vi "Configure Setpoint 1.vi"(5 "Retry Attempts (0)":i32 min=0, 7 "Unit Address (-1)":i32=-1, 8 "error in (no error)":errorcluster, 10 "Setpoint value":dbl format="%#_13g", 11 "VISA resource name (in)":refnum<visa-resource-name>) -> (0 "error out":errorcluster, 2 "Response Cluster":T1 {"Command ID" format="%x"}, 3 "VISA resource name (out)":refnum<visa-resource-name>)   [LabVIEW 2020, in "Omega Platinum Series.lvlib"]
doc: "Configures setpoint 1."
uses:
  <instrlib>/RxnRover/OmegaPlatinumSeriesDriver/Omega Platinum Series.lvlib
  <instrlib>/RxnRover/OmegaPlatinumSeriesDriver/Public/Type Defs/Response.ctl
panel:
  out "Command":string
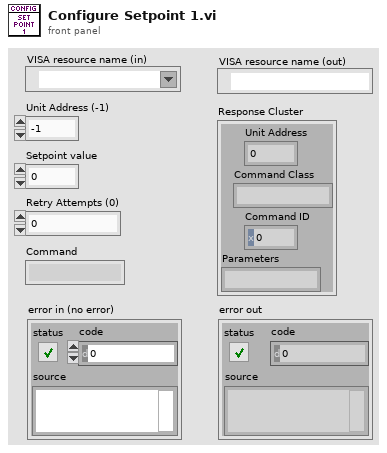
[diagram p1: front panel]
types:
  T1 = typedef "Omega Platinum Series.lvlib/Response.ctl" = cluster{"Unit Address":i32, "Command Class":string, "Command ID":u32, "Parameters":string}
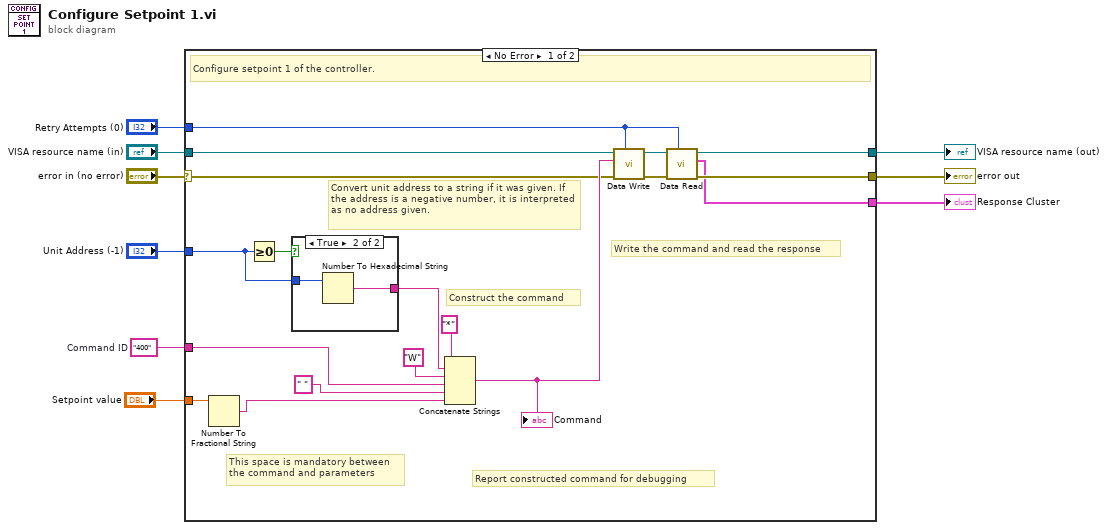
[diagram p0: block diagram]
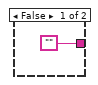
[diagram p2: hidden frame]
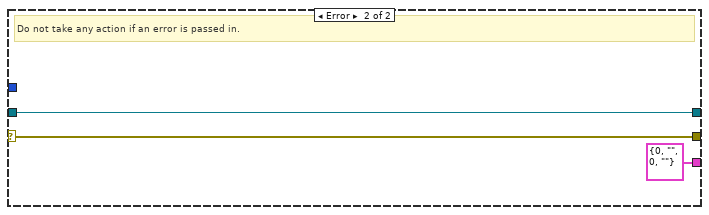
[diagram p3: hidden frame]
diagram:
  w9 = "400"  # Command ID
  n1 = case shown="No Error" "error in (no error)" {
    selector: "error in (no error)" -> [w21 w33]
    tunnel: w9 -> [w14 _]
    tunnel: "Unit Address (-1)" -> [w25 _]
    tunnel: [w17 w33] -> w6
    tunnel: "VISA resource name (in)" -> [w23 w32]
    tunnel: [w18 w32] -> w4
    tunnel: [w16 T1 {"Unit Address"=0, "Command Class"="", "Command ID"=0, "Parameters"=""} ("Response Cluster")] -> w3
    tunnel: "Setpoint value" -> [w12 _]
    tunnel: "Retry Attempts (0)" -> [w10 _]
    frame No Error {
      # "Report constructed command for debugging"
      # "Write the command and read the response"
      # "This space is mandatory between\nthe command and parameters"
      # "Convert unit address to a string if it was given. If the address is a negative number, it is interpreted as no address given."
      # "Construct the command"
      # "Configure setpoint 1 of the controller."
      n2 = Number To Fractional String(number=w12) -> (F-format string=w11:string)  [unwired: 3 in]
      n3 = Greater Or Equal To 0?(x=w25) -> (x >= 0?=w27:bool)
      n4 = case shown="True" w27 {
        tunnel: w25 -> [_ w30]
        tunnel: ["" w29] -> w24
        frame False {
        }
        frame True {
          n5 = Number To Hexadecimal String(2:w30) -> (0:w29:string)  [unwired: 1 in]
        }
      }
      n6 = Concatenate Strings("*" ("string"), w24, "W" ("string"), w14, " " ("string"), w11) -> (w22:string)
      "Command" <- w22
      n7 = call <instrlib>:"Data Write.vi"("Retry Attempts (0)"=w10, "error in (no error)"=w21, "Command"=w22, "VISA Refnum in"=w23) -> ("error out"=w20:errorcluster, "VISA Refnum out"=w19:refnum<visa-resource-name>)  [unwired: 6 in]
      n8 = call <instrlib>:"Data Read.vi"("Retry Attempts (0)"=w10, "error in (no error)"=w20, "VISA Refnum in"=w19) -> ("error out"=w17:errorcluster, "Response Cluster"=w16:T1, "VISA Refnum out"=w18:refnum<visa-resource-name>)  [unwired: 5 in, 1 out]
    }
    frame Error {
      # "Do not take any action if an error is passed in."
    }
  }
  "error out" <- w6
  "VISA resource name (out)" <- w4
  "Response Cluster" <- w3
